vi "Calculate Classic Gain.vi"(7 "Peak Indicies":i32[](array[numeric]), 8 "error in (no error)":errorcluster, 9 "Response in":dbl[][](array[numeric]), 10 "Stimulus in":dbl[][](array[numeric]), 11 "Head Impulse Fit in":refnum<class "Head Impulse Fit.lvclass">) -> (0 "error out":errorcluster, 1 "Response out":dbl[][](array[numeric]), 2 "Stimulus out":dbl[][](array[numeric]), 3 "Head Impulse Fit out":refnum<class "Head Impulse Fit.lvclass">)   [LabVIEW 2016, in "Head Impulse Fit.lvclass"]
uses:
  Head Impulse Fit.lvclass
  Head Impulse Fit.lvclass/Head Impulse Fit.ctl
  comm/stats/stats.lvlib
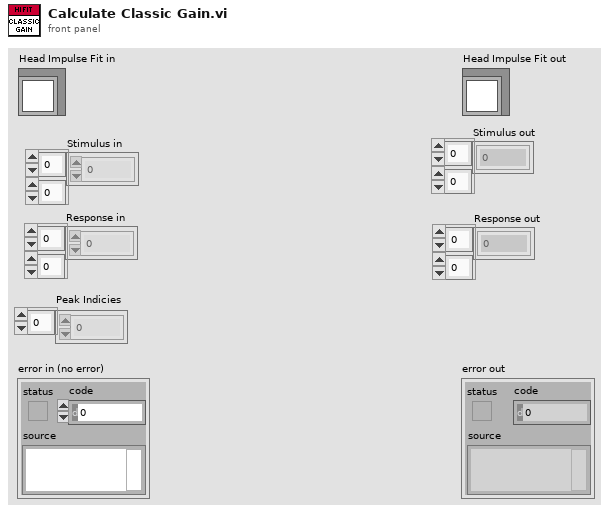
[diagram p1: front panel]
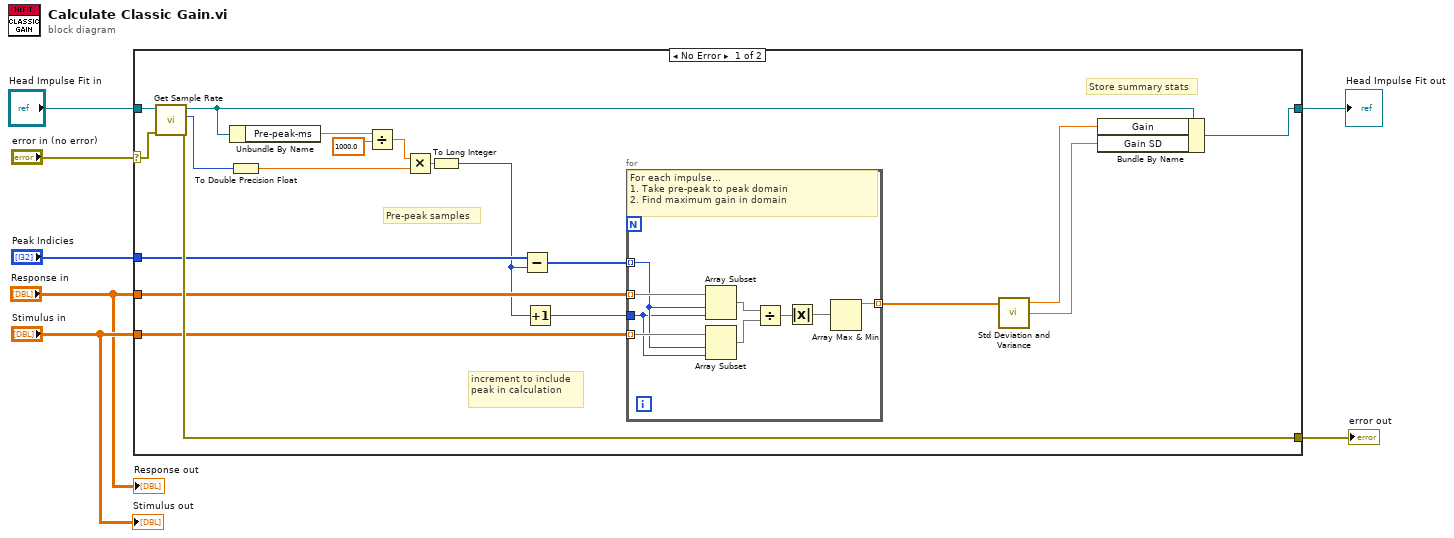
[diagram p0: block diagram]
diagram:
  n1 = case shown="No Error" "error in (no error)" {
    selector: "error in (no error)" -> [w24 w38]
    tunnel: [w27 w38] -> w6
    tunnel: [w17 w37] -> w4
    tunnel: "Head Impulse Fit in" -> [w25 w37]
    tunnel: "Peak Indicies" -> [w20 _]
    tunnel: "Stimulus in" -> [w21 _]
    tunnel: "Response in" -> [w22 _]
    frame No Error {
      # "increment to include peak in calculation"
      # "Store summary stats"
      # "Pre-peak samples"
      n2 = call-dynamic "Get Sample Rate.vi"("error in (no error)"=w24, "Abstract Fit in"=w25) -> ("error out"=w27:errorcluster, "Sample Rate"=w23:i32, "Abstract Fit out"=w18:refnum<class "Head Impulse Fit.lvclass">)  [unwired: 7 in]
      n3 = Unbundle By Name(w18) -> ("Pre-peak-ms"=w13:dbl)
      n4 = To Double Precision Float(number=w23) -> (double precision float=w11:dbl)
      n5 = Divide(x=w13, y=1000.0) -> (x/y=w12:dbl)
      n6 = Multiply(x=w12, y=w11) -> (x*y=w26:dbl)
      n7 = To Long Integer(number=w26) -> (32bit integer=w10:i32)
      n8 = Subtract(x=w20, y=w10) -> (x-y=w19:i32[])
      n9 = Increment(x=w10) -> (x+1=w9:i32)
      n10 = for {
        tunnel: [w36] -> w8 mode=indexing
        tunnel: w22 -> [w35] mode=indexing
        tunnel: w21 -> [w34] mode=indexing
        tunnel: w19 -> [w33] mode=indexing
        tunnel: w9 -> [w32]
        # "For each impulse...\n1. Take pre-peak to peak domain\n2. Find maximum gain in domain"
        n11 = Array Subset(array=w35, index=w33, length=w32) -> (w31:dbl[])
        n12 = Array Subset(array=w34, index=w33, length=w32) -> (w30:dbl[])
        n13 = Divide(x=w31, y=w30) -> (x/y=w29:dbl[])
        n14 = Absolute Value(x=w29) -> (abs(x)=w28:dbl[])
        n15 = Array Max & Min(array=w28) -> (max value=w36:dbl)  [unwired: 3 out]
      }
      n16 = call "Std Deviation and Variance.vi"("X"=w8) -> ("mean"=w16:dbl, "standard deviation"=w15:dbl)  [unwired: 1 in, 1 out]
      n17 = Bundle By Name(cluster=w18, "Gain"=w16, "Gain SD"=w15) -> (w17:refnum<class "Head Impulse Fit.lvclass">)
    }
    frame Error {
    }
  }
  "error out" <- w6
  "Head Impulse Fit out" <- w4
  "Stimulus out" <- "Stimulus in"
  "Response out" <- "Response in"
